vi "Run sprinkler.vi"(8 "error in (no error)":errorcluster, 11 "Application Data":T1={"Zone Indicators"={"North"=FALSE, "East"=FALSE, "South"=FALSE, "West"=FALSE, "Timing"=0.0}, "Controller Status"="", "Zone Setup Array"=[], "Sprinkler running"=FALSE, "Run Selector"=FALSE, "Current zone index"=0, "Suspended"=FALSE, "Water Pressure Sensor (%)"=11, "Rain"=FALSE} {"Water Pressure Sensor (%)" scale=0.0..100.0}) -> (0 "error out":errorcluster, 1 "Sprinkler running?":bool, 3 "Application Data 2":T1={"Zone Indicators"={"North"=FALSE, "East"=FALSE, "South"=FALSE, "West"=FALSE, "Timing"=0.0}, "Controller Status"="", "Zone Setup Array"=[], "Sprinkler running"=FALSE, "Run Selector"=FALSE, "Current zone index"=0, "Suspended"=FALSE, "Water Pressure Sensor (%)"=11, "Rain"=FALSE} {"Water Pressure Sensor (%)" scale=0.0..100.0})   [LabVIEW 2019]
doc: "This VI handles sprinkler operation and timing."
uses:
  Controls/Application Data.ctl
  Controls/Zone Indicators.ctl
  Controls/Controller Status.ctl
  Controls/Zone Setup Array.ctl
  Controls/Water Pressure Sensor.ctl
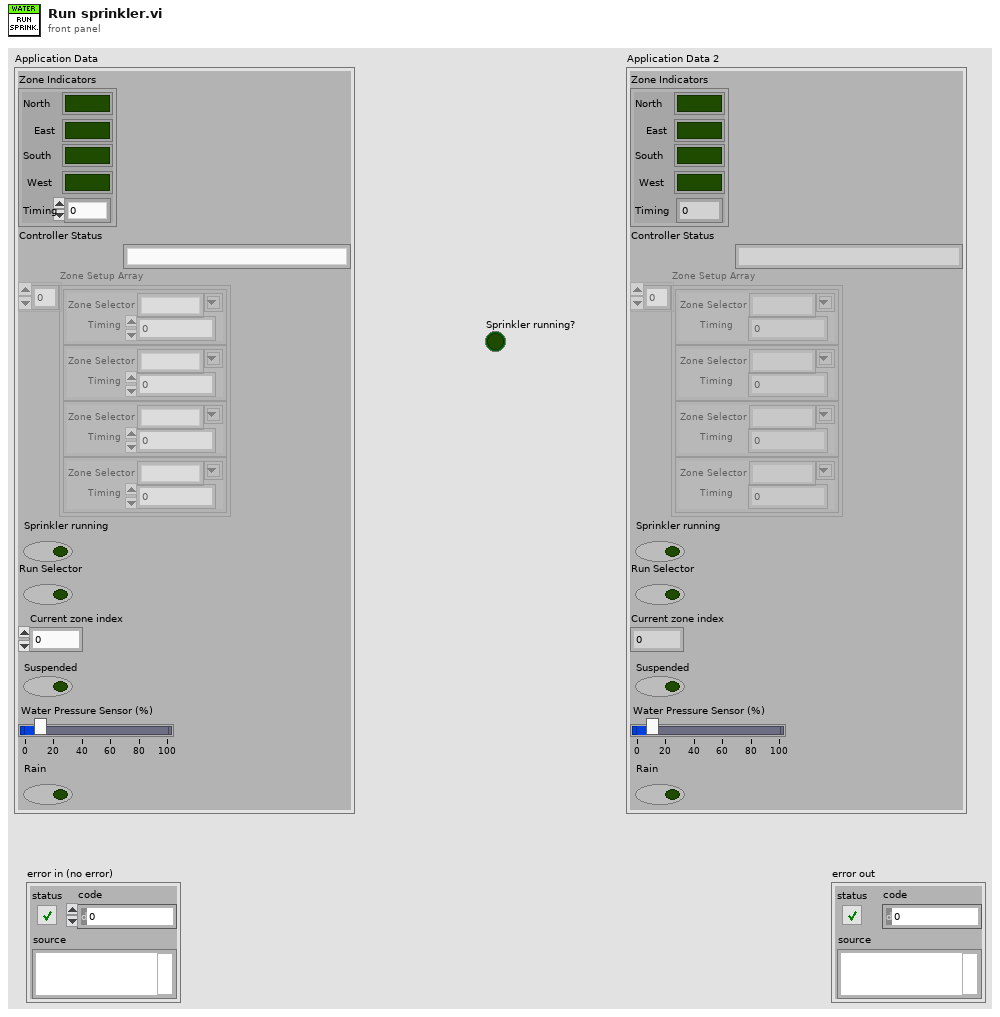
[diagram p1: front panel]
types:
  T1 = typedef "Application Data.ctl" = cluster{"Zone Indicators":T2, "Controller Status":T3, "Zone Setup Array":T4, "Sprinkler running":bool, "Run Selector":bool, "Current zone index":i32, "Suspended":bool, "Water Pressure Sensor (%)":T5, "Rain":bool}
  T2 = typedef "Zone Indicators.ctl" = cluster{"North":bool, "East":bool, "South":bool, "West":bool, "Timing":sgl}
  T3 = typedef "Controller Status.ctl" = string
  T4 = typedef "Zone Setup Array.ctl" = cluster{"Zone Selector":string, "Timing":dbl}[]
  T5 = typedef "Water Pressure Sensor.ctl" = u32
  T6 = enum16{"Get Time", "Reset Time", "Pause", "Resume"}
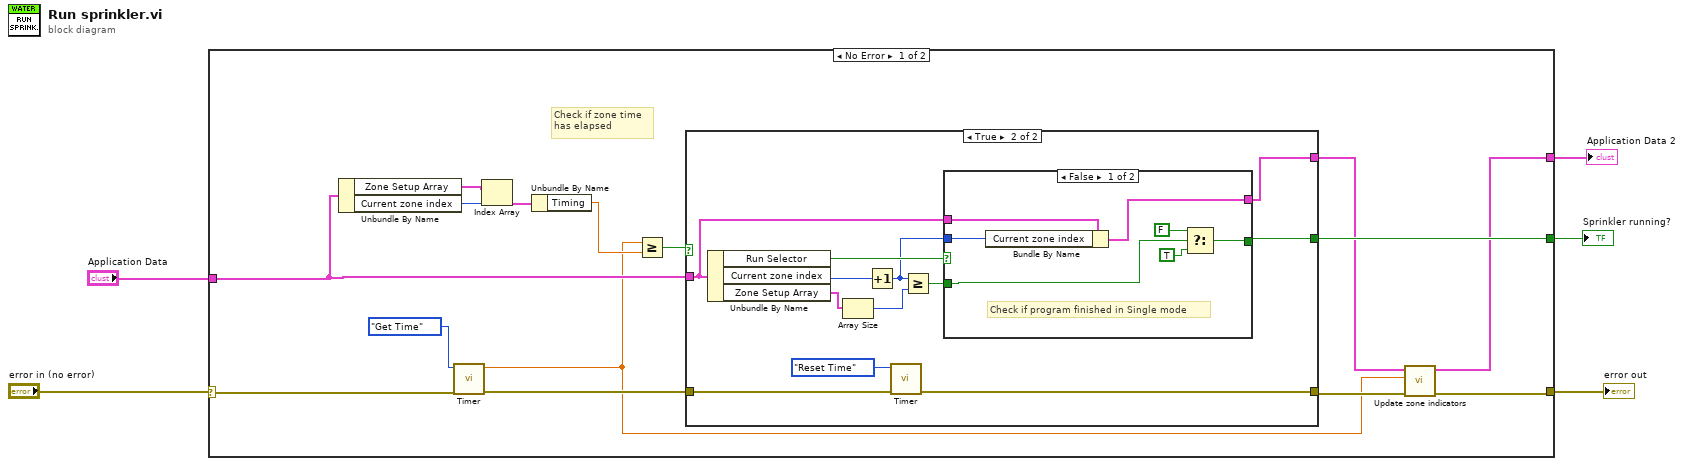
[diagram p0: block diagram]
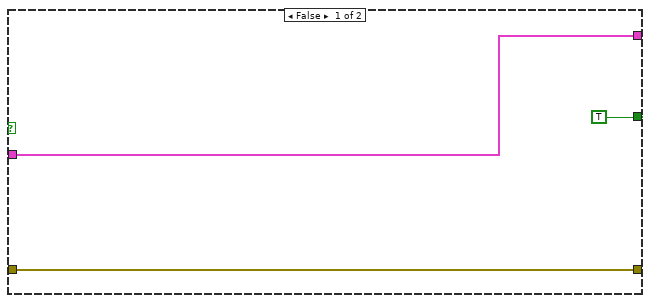
[diagram p2: hidden frame]
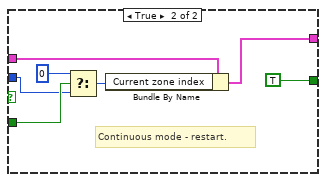
[diagram p3: hidden frame]
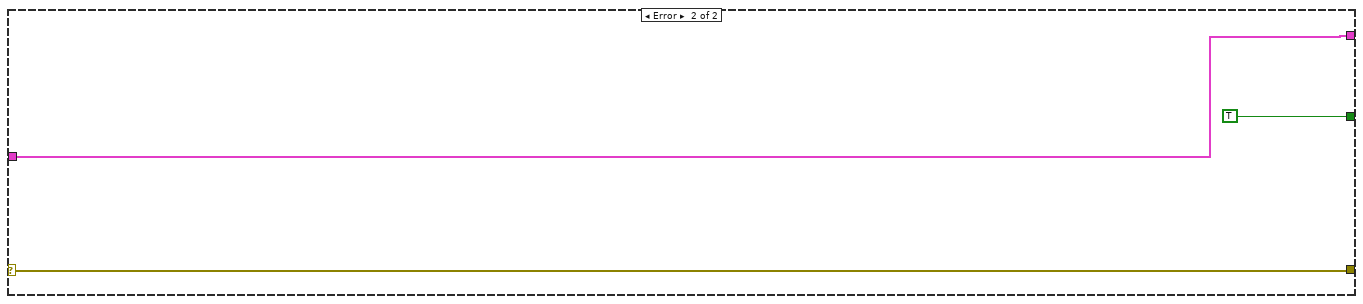
[diagram p4: hidden frame]
diagram:
  n1 = case shown="No Error" "error in (no error)" {
    selector: "error in (no error)" -> [w9 w52]
    tunnel: "Application Data" -> [w10 w51]
    tunnel: [w17 TRUE ("Program finished?")] -> w4
    tunnel: [w11 w52] -> w3
    tunnel: [w7 w51] -> w1
    frame No Error {
      # "Check if zone time\nhas elapsed"
      n2 = Unbundle By Name(w10) -> ("Zone Setup Array"=w16:T4, "Current zone index"=w15:i32)
      n3 = call "Timer.vi"("error in (no error)"=w9, "Enum"=T6."Get Time") -> ("error out"=w18:errorcluster, "Numeric"=w6:sgl)  [unwired: 8 in]
      n4 = Index Array(array=w16, index=w15) -> (element=w14:cluster{"Zone Selector":string, "Timing":dbl})
      n5 = Unbundle By Name(w14) -> ("Timing"=w13:dbl)
      n6 = Greater Or Equal?(x=w6, y=w13) -> (x >= y?=w19:bool)
      n7 = case shown="True" w19 {
        tunnel: w10 -> [w21 w26]
        tunnel: w18 -> [w22 w34]
        tunnel: [w22 w33] -> w12
        tunnel: [TRUE ("Program finished?") w28] -> w17
        tunnel: [w21 w27] -> w8
        frame False {
        }
        frame True {
          n8 = Unbundle By Name(w26) -> ("Run Selector"=w32:bool, "Current zone index"=w30:i32, "Zone Setup Array"=w29:T4)
          n9 = Array Size(array=w29) -> (size(s)=w31:i32)
          n10 = Increment(x=w30) -> (x+1=w24:i32)
          n11 = call "Timer.vi"("error in (no error)"=w34, "Enum"=T6."Reset Time") -> ("error out"=w33:errorcluster)  [unwired: 8 in, 1 out]
          n12 = Greater Or Equal?(x=w24, y=w31) -> (x >= y?=w25:bool)
          n13 = case shown="False" w32 {
            tunnel: w26 -> [w42 w49]
            tunnel: [w36 w48] -> w27
            tunnel: [w40 TRUE ("Program finished?")] -> w28
            tunnel: w25 -> [w39 w46]
            tunnel: w24 -> [w41 w43]
            frame False {
              # "Check if program finished in Single mode"
              n14 = Bundle By Name(cluster=w42, "Current zone index"=w41) -> (w36:T1)
              n15 = Select(t=FALSE, s=w39, f=TRUE) -> (s? t:f=w40:bool)
            }
            frame True {
              # "Continuous mode - restart."
              n16 = Select(t=0 ("Current zone index"), s=w46, f=w43) -> (s? t:f=w45:i32)
              n17 = Bundle By Name(cluster=w49, "Current zone index"=w45) -> (w48:T1)
            }
          }
        }
      }
      n18 = call "Update zone indicators.vi"("error in (no error)"=w12, "Zone Indicators.Timing"=w6, "Application Data in"=w8) -> ("error out"=w11:errorcluster, "Application Data out"=w7:T1)  [unwired: 7 in]
    }
    frame Error {
    }
  }
  "error out" <- w3
  "Application Data 2" <- w1
  "Sprinkler running?" <- w4
